vi "arangeIdx.vi"(8 "error in (no error)":errorcluster, 9 "Offset":i32, 10 "Number":i32, 11 "MatOper in":refnum<class "MatOper.lvclass">) -> (0 "error out":errorcluster, 2 "Idx Array":i32[](array[numeric]), 3 "MatOper out":refnum<class "MatOper.lvclass">)   [LabVIEW 2016, in "OfcFunc.lvlib" / "MatOper.lvclass"]
doc: "Get the index array from offset value to specified integer. The default value of offset is 0."
uses:
  MatOper.lvclass
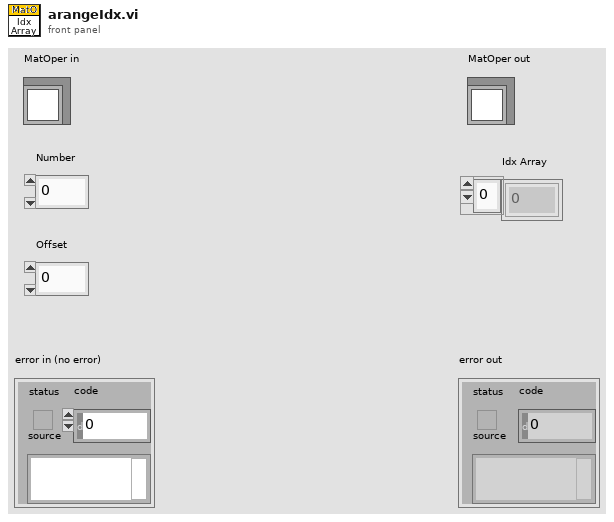
[diagram p1: front panel]
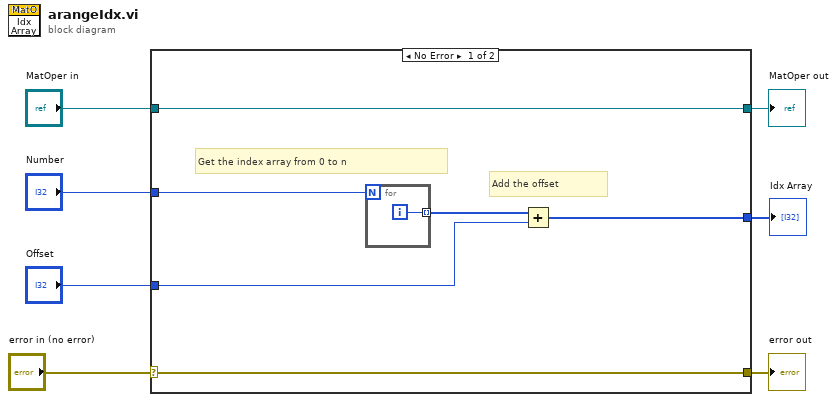
[diagram p0: block diagram]
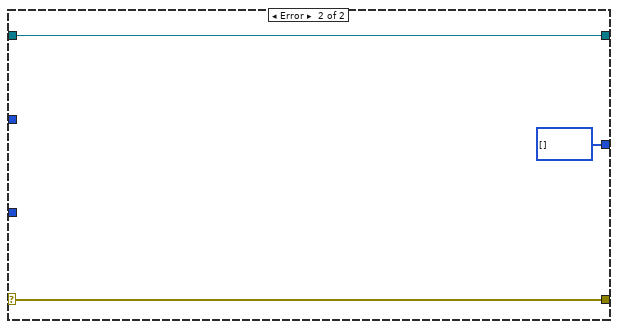
[diagram p2: hidden frame]
diagram:
  n1 = case shown="No Error" "error in (no error)" {
    selector: "error in (no error)" -> [w12 w17]
    tunnel: [w12 w17] -> w6
    tunnel: [w13 w16] -> w4
    tunnel: "MatOper in" -> [w13 w16]
    tunnel: [w10 i32[] []] -> w3
    tunnel: "Offset" -> [w9 _]
    tunnel: "Number" -> [w8 _]
    frame No Error {
      # "Add the offset"
      # "Get the index array from 0 to n"
      n2 = for {
        N: w8 -> [_]
        tunnel: [w14] -> w11 mode=indexing
        i -> [w14]
      }
      n3 = Add(x=w11, y=w9) -> (x+y=w10:i32[])
    }
    frame Error {
    }
  }
  "error out" <- w6
  "MatOper out" <- w4
  "Idx Array" <- w3
